vi "CoordinateConvert_CartesianToArm.vi"(3 "Wrist (rad)":dbl, 4 "Y (in)":dbl, 5 "X (in)":dbl) -> (0 "Wrist Angle (rad)":dbl, 1 "Radius (in)":dbl, 2 "Shoulder Angle (rad)":dbl)   [LabVIEW 2018]
uses:
  a1a48cbf-37a2-4001-9d38-1b405d9837cb.vi
  ArgosLib/ArgosLib.lvlib
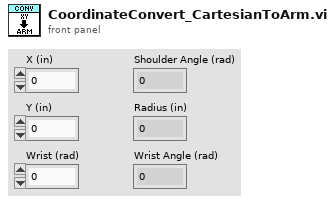
[diagram p1: front panel]
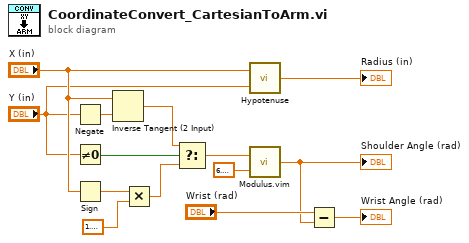
[diagram p0: block diagram]
diagram:
  n1 = Negate(x="Y (in)") -> (-x=w10:dbl)
  n2 = Not Equal To 0?(x="Y (in)") -> (x != 0?=w14:bool)
  n3 = Sign(1:"X (in)") -> (0:w13:dbl)
  n4 = Inverse Tangent (2 Input)(1:w10, 2:"X (in)") -> (0:w9:dbl)
  n5 = Multiply(x=w13, y=1.5707963267948966) -> (x*y=w11:dbl)
  n6 = Select(t=w9, s=w14, f=w11) -> (s? t:f=w8:dbl)
  n7 = call "Hypotenuse.vi"("Y"="Y (in)", "X"="X (in)") -> ("Hypotenuse"=→"Radius (in)":dbl)
  n8 = call "Modulus.vim"("y"=6.283185307179586, "x"=w8) -> ("x%y"=w2:dbl)
  "Shoulder Angle (rad)" <- w2
  n9 = Subtract(x="Wrist (rad)", y=w2) -> (x-y=→"Wrist Angle (rad)":dbl)
